vi "Area and time calculation_mains.vi"() -> ()   [LabVIEW 2014]
doc: "This example shows how to open, read, and display an AVI file in NI Vision. The VI reads the frames per second property and plays the images back at the rate specified by the AVI file."
uses:
  <vilib>/vision/NI_Vision_Development_Module.lvlib
panel:
  in  "Number of Erosion":i32=2
  in  "Low Pass/High Pass (Low)":bool
  out "t":dbl[][](array[numeric])
  out "s":dbl[][](array[numeric])
  in  "Info":bool
  in  "Binary":bool
  out "sum elements of array":dbl
  out "max value":dbl
  out "min value":dbl
  out "Error information":string
  out "Error of Velocity":dbl format="%#_4e"
  out "Velocity Mean":dbl format="%#_4e"
  out "Velocity\nArray":dbl[][](array[numeric])
  out "Y Step":sgl
  out "Num Final \nFrame":i32[](array[numeric])
  out "Num Initial\nFrame":i32[](array[numeric])
  in  "Velocity\nArray size":i32(slide)=3 scale=0.0..10.0
  in  "Range":cluster{"Lower value":sgl, "Upper value":sgl}={"Lower value"=0.0, "Upper value"=70.0}
  out "Initial Frame Pixel":dbl[](array[numeric])
  out "Initial Frame  Area":dbl[](array[numeric])
  out "Final Frame Area":dbl[](array[numeric])
  out "Final Frame Pixel":dbl[](array[numeric])
  out "pixel  value":dbl
  out "Area,µm^2":dbl
  in  "Si 2":T1={"X Size"=3, "Y Size"=3, "Order #"=4}
  out "appended array":i32[](array[numeric])
  out "dy":i32
  in  "Final Frame":i32(slide) scale=0.0..131.0
  in  "Initial Frame":i32(slide) scale=0.0..131.0
  out "time\nper frame":dbl
  in  "Frame":i32(slide) min=0 max=357 scale=0.0..131.0
  in  "Analyse":bool
  out "Image":T2(plugin-control)
  in  "stop":bool
  in  "Play":bool=TRUE
  # "White domain:\nRange 185-255"
  # "Black domain:\nRange 0-70"
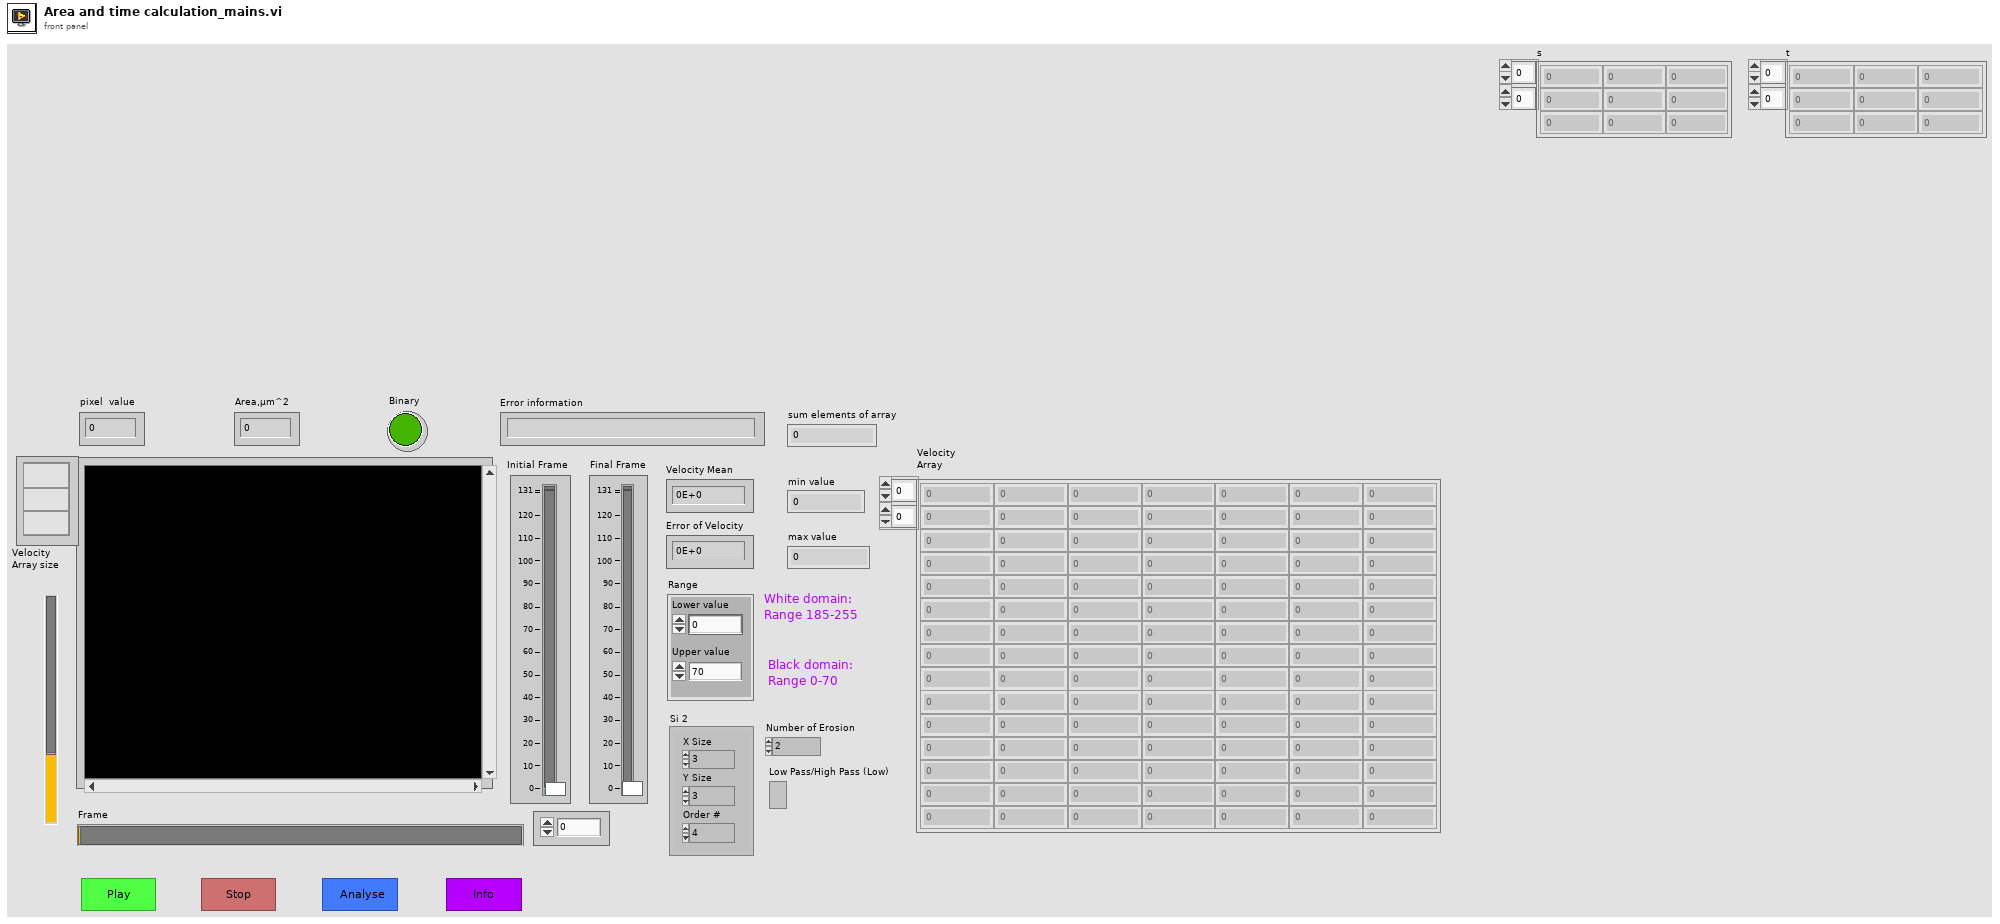
[diagram p1: front panel]
types:
  T1 = cluster{"X Size":i32, "Y Size":i32, "Order #":i32}
  T2 = typedef "IMAQ Image.ctl" = refnum<image>
  T3 = typedef "Image Type" = u32
  T4 = typedef "IMAQ AVI2 Refnum.ctl" = refnum<k20>
  T5 = cluster{"Width":u32, "Height":u32, "Frames Per Second":u32, "Codec":string, "Has Data":bool}
  T6 = typedef "Simple Grid Descriptor" = cluster{"X Step":sgl, "Y Step":sgl, "Unit":T7}
  T7 = typedef "Image Unit" = enum32{"Undefined", "Angström", "Micrometer", "Millimeter", "Centimeter", "Meter", "Kilometer", "Microinch", "Inch", "Feet", "Nautical miles", "Standard miles", "Steps"}
  T8 = cluster{"Global Rectangle":i32[], "Contours":cluster{"Contour Type":u32, "ROI Type":u32, "Points":i32[]}[]}
  T9 = typedef "IMAQ Rectangle" = cluster{"Left":i32, "Top":i32, "Right":i32, "Bottom":i32, "Rotation":dbl}
  T10 = typedef "Particle Parameters" = i32
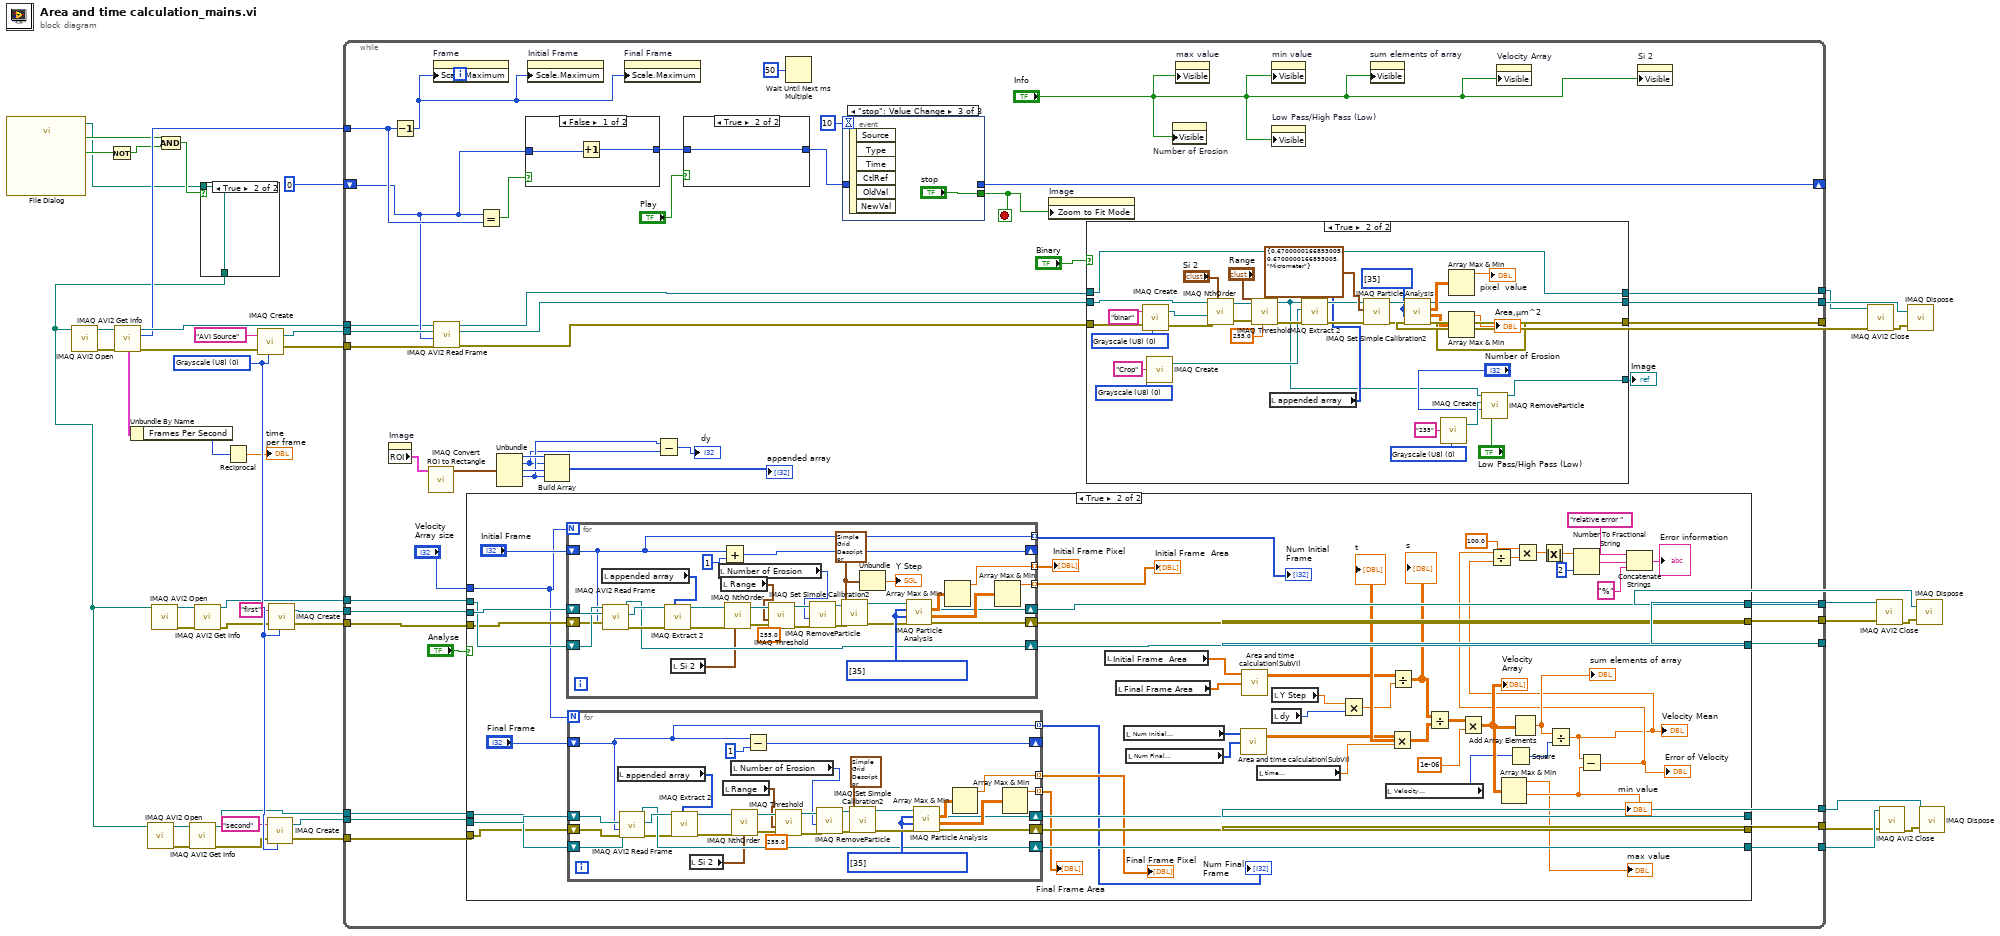
[diagram p0: block diagram]
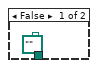
[diagram p2: hidden frame]
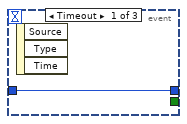
[diagram p4: hidden frame]
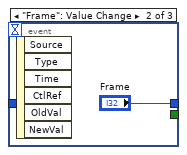
[diagram p5: hidden frame]
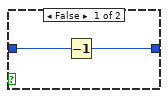
[diagram p7: hidden frame]
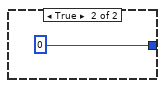
[diagram p8: hidden frame]
diagram:
  w37 = T3 0 items=["Grayscale (U8)", "Grayscale (I16)", "Grayscale (SGL)", "Complex (CSG)", "RGB (U32)", "HSL (U32)", "RGB (U64)", "Grayscale (U16)"] ("Image Type")
  n1 = call "File Dialog"() -> ("selected path"=w18:path, "exists"=w22:bool, "cancelled"=w21:bool)  [unwired: 12 in, 1 out]
  n2 = Not(x=w21) -> (.not. x?=w20:bool)
  n3 = Compound Arithmetic op=AND(w22, w20) -> (w19:bool)
  n4 = case shown="True" w19 {
    tunnel: w18 -> [_ w47]
    tunnel: [path "" ("selected path") w47] -> w6
    frame False {
    }
    frame True {
    }
  }
  n5 = call "IMAQ AVI2 Open"("AVI File Path"=w6) -> ("error out"=w45:errorcluster, "AVI Refnum"=w44:T4)  [unwired: 2 in, 7 out]
  n6 = call "IMAQ AVI2 Get Info"("error in (no error)"=w45, "AVI Refnum"=w44) -> ("error out"=w43:errorcluster, "Number of Frames"=w39:u32, "AVI Refnum (duplicate)"=w40:T4, "Frame Data"=w25:T5)  [unwired: 6 out]
  n7 = Unbundle By Name(w25) -> ("Frames Per Second"=w24:u32)
  n8 = call "IMAQ AVI2 Open"("AVI File Path"=w6) -> ("error out"=w33:errorcluster, "AVI Refnum"=w31:T4)  [unwired: 2 in, 7 out]
  n9 = call "IMAQ AVI2 Open"("AVI File Path"=w6) -> ("error out"=w34:errorcluster, "AVI Refnum"=w32:T4)  [unwired: 2 in, 7 out]
  n10 = call "IMAQ AVI2 Get Info"("error in (no error)"=w33, "AVI Refnum"=w31) -> ("error out"=w28:errorcluster, "AVI Refnum (duplicate)"=w16:T4)  [unwired: 8 out]
  n11 = call "IMAQ AVI2 Get Info"("error in (no error)"=w34, "AVI Refnum"=w32) -> ("error out"=w27:errorcluster, "AVI Refnum (duplicate)"=w26:T4)  [unwired: 8 out]
  n12 = Reciprocal(x=w24) -> (1/x=→"time\nper frame":dbl)
  n13 = call "IMAQ Create"("Image Name"="AVI Source", "Image Type"=w37, "error in (no error)"=w43) -> ("New Image"=w41:T2, "error out"=w42:errorcluster)  [unwired: 1 in, 1 out]
  n14 = call "IMAQ Create"("Image Name"="second", "Image Type"=w37, "error in (no error)"=w28) -> ("New Image"=w35:T2, "error out"=w15:errorcluster)  [unwired: 1 in, 1 out]
  n15 = call "IMAQ Create"("Image Name"="first", "Image Type"=w37, "error in (no error)"=w27) -> ("New Image"=w36:T2, "error out"=w14:errorcluster)  [unwired: 1 in, 1 out]
  n16 = while {
    tunnel: w41 -> [w91]
    tunnel: [w60] -> w1
    tunnel: w42 -> [w89]
    tunnel: w40 -> [w65]
    tunnel: w39 -> [w83]
    tunnel: w36 -> [w55]
    tunnel: w35 -> [w53]
    tunnel: w26 -> [w56]
    shift-right: [w84] -> _
    shift-left: u32 0 -> [w77]
    tunnel: w16 -> [w54]
    tunnel: w15 -> [w52]
    tunnel: w14 -> [w57]
    tunnel: [w76] -> w13
    tunnel: [w70] -> w12
    tunnel: [w69] -> w2
    tunnel: [w75] -> w11
    tunnel: [w74] -> w10
    tunnel: [w73] -> w8
    tunnel: [w63] -> w4
    tunnel: [w64] -> w3
    stop <- w66 stop-if-true
    n17 = property on="Image" class="ImageControl"() -> ("ROI"=w81:T8)  [unwired: 2 in, 2 out]
    n18 = Decrement(x=w83) -> (x-1=w58:u32)
    n19 = call "IMAQ Convert ROI to Rectangle"("ROI Descriptor"=w81) -> ("Rectangle"=w78:T9)  [unwired: 8 in, 1 out]
    n20 = property on="Frame" class="Slide (strict)"("Scale.Maximum"=w58) -> ()  [unwired: 2 in, 2 out]
    n21 = call "IMAQ AVI2 Read Frame"("error in (no error)"=w89, "Frame Number"=w77, "Image"=w91, "AVI Refnum"=w65) -> ("error out"=w49:errorcluster, "Image Out"=w50:T2, "AVI Refnum (duplicate)"=w51:T4)  [unwired: 5 out]
    n22 = case shown="True" "Analyse" {
      tunnel: w55 -> [w138 w192]
      tunnel: w53 -> [w136 w191]
      tunnel: w56 -> [w140 w190]
      tunnel: w54 -> [w137 w189]
      tunnel: w52 -> [w135 w188]
      tunnel: w57 -> [w139 w187]
      tunnel: [w140 w186] -> w76
      tunnel: [w138 w185] -> w70
      tunnel: [w136 w184] -> w69
      tunnel: [w137 w183] -> w75
      tunnel: [w135 w182] -> w74
      tunnel: [w139 w181] -> w73
      tunnel: "Velocity\nArray size" -> [_ w174]
      frame False {
      }
      frame True {
        n23 = for {
          N: w174 -> [_]
          shift-right: [w241] -> w185
          shift-left: w192 -> [w257]
          shift-right: [w242] -> w186
          shift-left: w190 -> [w256]
          shift-right: [w240] -> w181
          shift-left: w187 -> [w255]
          shift-right: [w234] -> _
          shift-left: "Initial Frame" -> [w233]
          tunnel: [w238] -> w176 mode=indexing
          tunnel: [w237] -> w175 mode=indexing
          tunnel: [w233] -> w161 mode=indexing
          w230 = T6 {"X Step"=0.67, "Y Step"=0.67, "Unit"=enum."Undefined"} ("Pixel Distances")
          w254 = T10[] [35] items=["Center of Mass X", "Center of Mass Y", "First Pixel X", "First Pixel Y", "Bounding Rect Left", "Bounding Rect Top", "Bounding Rect Right", "Bounding Rect Bottom", "Max Feret Diameter Start X", "Max Feret Diameter Start Y", "Max Feret Diameter End X", "Max Feret Diameter End Y", "Max Horiz. Segment Length Left", "Max Horiz. Segment Length Right", "Max Horiz. Segment Length Row", "-", "Bounding Rect Width", "Bounding Rect Height", "Bounding Rect Diagonal", "Perimeter", "Convex Hull Perimeter", "Holes' Perimeter", "Max Feret Diameter", "Equivalent Ellipse Major Axis", "Equivalent Ellipse Minor Axis", "Equivalent Ellipse Minor Axis (Feret)", "Equivalent Rect Long Side", "Equivalent Rect Short Side", "Equivalent Rect Diagonal", "Equivalent Rect Short Side (Feret)", "Average Horiz. Segment Length", "Average Vert. Segment Length", "Hydraulic Radius", "Waddel Disk Diameter", "-", "Area", "Holes' Area", "Particle & Holes' Area", "Convex Hull Area", "Image Area", "-", "Number of Holes", "Number of Horiz. Segments", "Number of Vert. Segments", "-", "Orientation", "Max Feret Diameter Orientation", "-", "% Area/Image Area", "% Area/(Particle & Holes' Area)", "Ratio of Equivalent Ellipse Axes", "Ratio of Equivalent Rect Sides", "-", "Elongation Factor", "Compactness Factor", "Heywood Circularity Factor", "Type Factor", "-", "Sum X", "Sum Y", "Sum XX", "Sum XY", "Sum YY", "Sum XXX", "Sum XXY", "Sum XYY", "Sum YYY", "-", "Moment of Inertia XX", "Moment of Inertia XY", "Moment of Inertia YY", "Moment of Inertia XXX", "Moment of Inertia XXY", "Moment of Inertia XYY", "Moment of Inertia YYY", "Norm. Moment of Inertia XX", "Norm. Moment of Inertia XY", "Norm. Moment of Inertia YY", "Norm. Moment of Inertia XXX", "Norm. Moment of Inertia XXY", "Norm. Moment of Inertia XYY", "Norm. Moment of Inertia YYY", "Hu Moment 1", "Hu Moment 2", "Hu Moment 3", "Hu Moment 4", "Hu Moment 5", "Hu Moment 6", "Hu Moment 7"] ("Pixel Measurements")
          n24 = local read "appended array"() -> (w235:i32[])
          n25 = call "IMAQ AVI2 Read Frame"("error in (no error)"=w255, "Frame Number"=w233, "Image"=w257, "AVI Refnum"=w256) -> ("error out"=w245:errorcluster, "Image Out"=w249:T2, "AVI Refnum (duplicate)"=w242:T4)  [unwired: 5 out]
          n26 = call "IMAQ Extract 2"("Optional Rectangle"=w235, "error in (no error)"=w245, "Image Src"=w249) -> ("error out"=w244:errorcluster, "Image Dst Out"=w248:T2)  [unwired: 7 in]
          n27 = local read "Si 2"() -> (w236:T1)
          n28 = local read "Number of Erosion"() -> (w225:i32)
          n29 = local read "Range"() -> (w231:cluster{"Lower value":sgl, "Upper value":sgl})
          n30 = Add(x=w233, y=1) -> (x+y=w234:i32)
          n31 = call "IMAQ NthOrder"("Image Src"=w248, "Size & Order #"=w236, "error in (no error)"=w244) -> ("Image Dst Out"=w247:T2, "error out"=w252:errorcluster)  [unwired: 4 in]
          n32 = call "IMAQ Threshold"("Replace Value"=sgl 255.0, "error in (no error)"=w252, "Range"=w231, "Image Src"=w247) -> ("error out"=w227:errorcluster, "Image Dst Out"=w229:T2)  [unwired: 6 in]
          n33 = call "IMAQ RemoveParticle"("error in (no error)"=w227, "Number of Erosion"=w225, "Image Src"=w229) -> ("error out"=w226:errorcluster, "Image Dst Out"=w228:T2)  [unwired: 7 in]
          n34 = call "IMAQ Set Simple Calibration2"("error in (no error)"=w226, "Pixel Distances"=w230, "Image"=w228) -> ("error out"=w243:errorcluster, "Calibration Template Image"=w246:T2)  [unwired: 7 in]
          n35 = Unbundle(w230) -> ("Y Step"=→"Y Step":sgl)  [unwired: 2 out]
          n36 = call "IMAQ Particle Analysis"("error in (no error)"=w243, "Real-World Measurements"=w254, "Pixel Measurements"=w254, "Image"=w246) -> ("error out"=w240:errorcluster, "Particle Measurements (Real-World)"=w250:dbl[][], "Particle Measurements (Pixels)"=w251:dbl[][], "Image Out (duplicate)"=w241:T2)  [unwired: 2 in, 2 out]
          n37 = Array Max & Min(array=w251) -> (max value=w238:dbl)  [unwired: 3 out]
          n38 = Array Max & Min(array=w250) -> (max value=w237:dbl)  [unwired: 3 out]
        }
        "Initial Frame Pixel" <- w176
        "Initial Frame  Area" <- w175
        "Num Initial\nFrame" <- w161
        n39 = for {
          N: w174 -> [_]
          shift-right: [w210] -> w184
          shift-left: w191 -> [w224]
          shift-right: [w209] -> w183
          shift-left: w189 -> [w223]
          shift-right: [w201] -> _
          shift-left: "Final Frame" -> [w200]
          tunnel: [w205] -> w178 mode=indexing
          tunnel: [w204] -> w177 mode=indexing
          shift-right: [w208] -> w182
          shift-left: w188 -> [w222]
          tunnel: [w200] -> w160 mode=indexing
          w212 = T10[] [35] items=["Center of Mass X", "Center of Mass Y", "First Pixel X", "First Pixel Y", "Bounding Rect Left", "Bounding Rect Top", "Bounding Rect Right", "Bounding Rect Bottom", "Max Feret Diameter Start X", "Max Feret Diameter Start Y", "Max Feret Diameter End X", "Max Feret Diameter End Y", "Max Horiz. Segment Length Left", "Max Horiz. Segment Length Right", "Max Horiz. Segment Length Row", "-", "Bounding Rect Width", "Bounding Rect Height", "Bounding Rect Diagonal", "Perimeter", "Convex Hull Perimeter", "Holes' Perimeter", "Max Feret Diameter", "Equivalent Ellipse Major Axis", "Equivalent Ellipse Minor Axis", "Equivalent Ellipse Minor Axis (Feret)", "Equivalent Rect Long Side", "Equivalent Rect Short Side", "Equivalent Rect Diagonal", "Equivalent Rect Short Side (Feret)", "Average Horiz. Segment Length", "Average Vert. Segment Length", "Hydraulic Radius", "Waddel Disk Diameter", "-", "Area", "Holes' Area", "Particle & Holes' Area", "Convex Hull Area", "Image Area", "-", "Number of Holes", "Number of Horiz. Segments", "Number of Vert. Segments", "-", "Orientation", "Max Feret Diameter Orientation", "-", "% Area/Image Area", "% Area/(Particle & Holes' Area)", "Ratio of Equivalent Ellipse Axes", "Ratio of Equivalent Rect Sides", "-", "Elongation Factor", "Compactness Factor", "Heywood Circularity Factor", "Type Factor", "-", "Sum X", "Sum Y", "Sum XX", "Sum XY", "Sum YY", "Sum XXX", "Sum XXY", "Sum XYY", "Sum YYY", "-", "Moment of Inertia XX", "Moment of Inertia XY", "Moment of Inertia YY", "Moment of Inertia XXX", "Moment of Inertia XXY", "Moment of Inertia XYY", "Moment of Inertia YYY", "Norm. Moment of Inertia XX", "Norm. Moment of Inertia XY", "Norm. Moment of Inertia YY", "Norm. Moment of Inertia XXX", "Norm. Moment of Inertia XXY", "Norm. Moment of Inertia XYY", "Norm. Moment of Inertia YYY", "Hu Moment 1", "Hu Moment 2", "Hu Moment 3", "Hu Moment 4", "Hu Moment 5", "Hu Moment 6", "Hu Moment 7"] ("Pixel Measurements")
          n40 = local read "appended array"() -> (w202:i32[])
          n41 = call "IMAQ AVI2 Read Frame"("error in (no error)"=w222, "Frame Number"=w200, "Image"=w224, "AVI Refnum"=w223) -> ("error out"=w207:errorcluster, "Image Out"=w211:T2, "AVI Refnum (duplicate)"=w209:T4)  [unwired: 5 out]
          n42 = call "IMAQ Extract 2"("Optional Rectangle"=w202, "error in (no error)"=w207, "Image Src"=w211) -> ("error out"=w220:errorcluster, "Image Dst Out"=w217:T2)  [unwired: 7 in]
          n43 = local read "Si 2"() -> (w203:T1)
          n44 = local read "Range"() -> (w199:cluster{"Lower value":sgl, "Upper value":sgl})
          n45 = local read "Number of Erosion"() -> (w193:i32)
          n46 = call "IMAQ NthOrder"("Image Src"=w217, "Size & Order #"=w203, "error in (no error)"=w220) -> ("Image Dst Out"=w218:T2, "error out"=w214:errorcluster)  [unwired: 4 in]
          n47 = Subtract(x=w200, y=1) -> (x-y=w201:i32)
          n48 = call "IMAQ Threshold"("Replace Value"=sgl 255.0, "error in (no error)"=w214, "Range"=w199, "Image Src"=w218) -> ("error out"=w197:errorcluster, "Image Dst Out"=w196:T2)  [unwired: 6 in]
          n49 = call "IMAQ RemoveParticle"("error in (no error)"=w197, "Number of Erosion"=w193, "Image Src"=w196) -> ("error out"=w194:errorcluster, "Image Dst Out"=w195:T2)  [unwired: 7 in]
          n50 = call "IMAQ Set Simple Calibration2"("error in (no error)"=w194, "Pixel Distances"=T6 {"X Step"=0.67, "Y Step"=0.67, "Unit"=enum."Micrometer"}, "Image"=w195) -> ("error out"=w221:errorcluster, "Calibration Template Image"=w219:T2)  [unwired: 7 in]
          n51 = call "IMAQ Particle Analysis"("error in (no error)"=w221, "Real-World Measurements"=w212, "Pixel Measurements"=w212, "Image"=w219) -> ("error out"=w208:errorcluster, "Particle Measurements (Real-World)"=w216:dbl[][], "Particle Measurements (Pixels)"=w215:dbl[][], "Image Out (duplicate)"=w210:T2)  [unwired: 2 in, 2 out]
          n52 = Array Max & Min(array=w215) -> (max value=w205:dbl)  [unwired: 3 out]
          n53 = Array Max & Min(array=w216) -> (max value=w204:dbl)  [unwired: 3 out]
        }
        "Final Frame Pixel" <- w178
        "Final Frame Area" <- w177
        "Num Final \nFrame" <- w160
        n54 = local read "Initial Frame  Area"() -> (w142:dbl[])
        n55 = local read "Final Frame Area"() -> (w143:dbl[])
        n56 = local read "Num Initial\nFrame"() -> (w162:i32[])
        n57 = local read "Num Final \nFrame"() -> (w163:i32[])
        n58 = call "Area and time calculation(SubVI).vi"("Array in 2"=w163, "Array in"=w162) -> ("Array out"=w164:dbl[][])  [unwired: 2 in]
        n59 = call "Area and time calculation(SubVI).vi"("Array in 2"=w143, "Array in"=w142) -> ("Array out"=w168:dbl[][])  [unwired: 2 in]
        n60 = local read "time\nper frame"() -> (w165:dbl)
        n61 = local read "Y Step"() -> (w166:sgl)
        n62 = local read "dy"() -> (w167:i32)
        n63 = Multiply(x=w166, y=w167) -> (x*y=w169:sgl)
        n64 = local read "Velocity\nArray size"() -> (w149:i32)
        n65 = Multiply(x=w164, y=w165) -> (x*y=w171:dbl[][])
        "t" <- w171
        n66 = Divide(x=w168, y=w169) -> (x/y=w170:dbl[][])
        "s" <- w170
        n67 = Divide(x=w170, y=w171) -> (x/y=w172:dbl[][])
        n68 = Multiply(x=w172, y=1e-06) -> (x*y=w159:dbl[][])
        "Velocity\nArray" <- w159
        n69 = Array Max & Min(array=w159) -> (max value=→"max value":dbl, min value=w157:dbl)  [unwired: 2 out]
        "min value" <- w157
        n70 = Square(x=w149) -> (x^2=w148:i32)
        n71 = Add Array Elements(numeric array=w159) -> (sum=w158:dbl)
        "sum elements of array" <- w158
        n72 = Divide(x=w158, y=w148) -> (x/y=w146:dbl)
        "Velocity Mean" <- w146
        n73 = Subtract(x=w146, y=w157) -> (x-y=w147:dbl)
        "Error of Velocity" <- w147
        n74 = Divide(x=w147, y=w146) -> (x/y=w156:dbl)
        n75 = Multiply(x=100.0, y=w156) -> (x*y=w145:dbl)
        n76 = Absolute Value(x=w145) -> (abs(x)=w144:dbl)
        n77 = Number To Fractional String(number=w144, precision (6)=i16 2) -> (F-format string=w154:string)  [unwired: 2 in]
        n78 = Concatenate Strings("relative error " ("string"), w154, "%" ("string")) -> (→"Error information":string)
      }
    }
    n79 = Equal?(x=w77, y=w83) -> (x = y?=w92:bool)
    n80 = Unbundle(w78) -> ("Left"=w80:i32, "Top"=w67:i32, "Right"=w79:i32, "Bottom"=w68:i32)  [unwired: 1 out]
    n81 = case shown="False" w92 {
      tunnel: w77 -> [w262 _]
      tunnel: [w261 i16 0] -> w86
      frame False {
        n82 = Increment(x=w262) -> (x+1=w261:u32)
      }
      frame True {
      }
    }
    n83 = property on="Initial Frame" class="Slide (strict)"("Scale.Maximum"=w58) -> ()  [unwired: 2 in, 2 out]
    n84 = Build Array(w80, w67, w79, w68) -> (→"appended array":i32[])
    n85 = property on="Final Frame" class="Slide (strict)"("Scale.Maximum"=w58) -> ()  [unwired: 2 in, 2 out]
    n86 = Subtract(x=w68, y=w67) -> (x-y=→"dy":i32)
    n87 = case shown="True" "Play" {
      tunnel: w86 -> [w259 w260]
      tunnel: [w258 w260] -> w85
      frame False {
        n88 = Decrement(x=w259) -> (x-1=w258:u32)
      }
      frame True {
      }
    }
    n89 = Wait Until Next ms Multiple(millisecond multiple=u32 50) -> ()  [unwired: 1 out]
    n90 = event shown="[2] \"stop\": Value Change" {
      selector: _ -> [_ _ _]
      dyn-events: _ -> [_ _ _]
      timeout: 10 -> [_ _ _]
      tunnel: w85 -> [w132 _ _]
      tunnel: [w132 "Frame" _] -> w84
      tunnel: [_ _ "stop"] -> w66
      event Timeout {
        n91 = event-data() -> ()  [unwired: 1 in, 3 out]
      }
      event "Frame": Value Change {
        n92 = event-data() -> ()  [unwired: 1 in, 6 out]
      }
      event "stop": Value Change {
        n93 = event-data() -> ()  [unwired: 1 in, 6 out]
      }
    }
    n94 = property on="Image" class="ImageControl"("Zoom to Fit Mode"=w66) -> ()  [unwired: 2 in, 2 out]
    n95 = case shown="True" "Binary" {
      tunnel: w51 -> [w95 w117]
      tunnel: [w95 w117] -> w60
      tunnel: w49 -> [w94 w128]
      tunnel: w50 -> [w93 w111]
      tunnel: [w93 w118] -> w63
      tunnel: [w94 w114] -> w64
      tunnel: [w93 w102] -> w61
      frame False {
      }
      frame True {
        w97 = T3 0 items=["Grayscale (U8)", "Grayscale (I16)", "Grayscale (SGL)", "Complex (CSG)", "RGB (U32)", "HSL (U32)", "RGB (U64)", "Grayscale (U16)"] ("Image Type")
        w104 = T3 0 items=["Grayscale (U8)", "Grayscale (I16)", "Grayscale (SGL)", "Complex (CSG)", "RGB (U32)", "HSL (U32)", "RGB (U64)", "Grayscale (U16)"] ("Image Type")
        w121 = T10[] [35] items=["Center of Mass X", "Center of Mass Y", "First Pixel X", "First Pixel Y", "Bounding Rect Left", "Bounding Rect Top", "Bounding Rect Right", "Bounding Rect Bottom", "Max Feret Diameter Start X", "Max Feret Diameter Start Y", "Max Feret Diameter End X", "Max Feret Diameter End Y", "Max Horiz. Segment Length Left", "Max Horiz. Segment Length Right", "Max Horiz. Segment Length Row", "-", "Bounding Rect Width", "Bounding Rect Height", "Bounding Rect Diagonal", "Perimeter", "Convex Hull Perimeter", "Holes' Perimeter", "Max Feret Diameter", "Equivalent Ellipse Major Axis", "Equivalent Ellipse Minor Axis", "Equivalent Ellipse Minor Axis (Feret)", "Equivalent Rect Long Side", "Equivalent Rect Short Side", "Equivalent Rect Diagonal", "Equivalent Rect Short Side (Feret)", "Average Horiz. Segment Length", "Average Vert. Segment Length", "Hydraulic Radius", "Waddel Disk Diameter", "-", "Area", "Holes' Area", "Particle & Holes' Area", "Convex Hull Area", "Image Area", "-", "Number of Holes", "Number of Horiz. Segments", "Number of Vert. Segments", "-", "Orientation", "Max Feret Diameter Orientation", "-", "% Area/Image Area", "% Area/(Particle & Holes' Area)", "Ratio of Equivalent Ellipse Axes", "Ratio of Equivalent Rect Sides", "-", "Elongation Factor", "Compactness Factor", "Heywood Circularity Factor", "Type Factor", "-", "Sum X", "Sum Y", "Sum XX", "Sum XY", "Sum YY", "Sum XXX", "Sum XXY", "Sum XYY", "Sum YYY", "-", "Moment of Inertia XX", "Moment of Inertia XY", "Moment of Inertia YY", "Moment of Inertia XXX", "Moment of Inertia XXY", "Moment of Inertia XYY", "Moment of Inertia YYY", "Norm. Moment of Inertia XX", "Norm. Moment of Inertia XY", "Norm. Moment of Inertia YY", "Norm. Moment of Inertia XXX", "Norm. Moment of Inertia XXY", "Norm. Moment of Inertia XYY", "Norm. Moment of Inertia YYY", "Hu Moment 1", "Hu Moment 2", "Hu Moment 3", "Hu Moment 4", "Hu Moment 5", "Hu Moment 6", "Hu Moment 7"] ("Pixel Measurements")
        w129 = T3 0 items=["Grayscale (U8)", "Grayscale (I16)", "Grayscale (SGL)", "Complex (CSG)", "RGB (U32)", "HSL (U32)", "RGB (U64)", "Grayscale (U16)"] ("Image Type")
        n96 = call "IMAQ Create"("Image Name"="binar", "Image Type"=w129, "error in (no error)"=w128) -> ("New Image"=w112:T2, "error out"=w110:errorcluster)  [unwired: 1 in, 1 out]
        n97 = call "IMAQ Create"("Image Name"="Crop", "Image Type"=w104) -> ("New Image"=w103:T2)  [unwired: 2 in, 2 out]
        n98 = call "IMAQ NthOrder"("Image Src"=w111, "Size & Order #"="Si 2", "Image Dst"=w112, "error in (no error)"=w110) -> ("Image Dst Out"=w131:T2, "error out"=w127:errorcluster)  [unwired: 3 in]
        n99 = call "IMAQ Threshold"("Replace Value"=sgl 255.0, "error in (no error)"=w127, "Range"="Range", "Image Src"=w131) -> ("error out"=w109:errorcluster, "Image Dst Out"=w96:T2)  [unwired: 6 in]
        n100 = local read "appended array"() -> (w106:i32[])
        n101 = call "IMAQ Extract 2"("Optional Rectangle"=w106, "error in (no error)"=w109, "Image Dst"=w103, "Image Src"=w96) -> ("error out"=w108:errorcluster, "Image Dst Out"=w107:T2)  [unwired: 6 in]
        n102 = call "IMAQ Set Simple Calibration2"("error in (no error)"=w108, "Pixel Distances"=T6 {"X Step"=0.67, "Y Step"=0.67, "Unit"=enum."Micrometer"}, "Image"=w107) -> ("error out"=w123:errorcluster, "Calibration Template Image"=w122:T2)  [unwired: 7 in]
        n103 = call "IMAQ Particle Analysis"("error in (no error)"=w123, "Real-World Measurements"=w121, "Pixel Measurements"=w121, "Image"=w122) -> ("error out"=w114:errorcluster, "Particle Measurements (Real-World)"=w119:dbl[][], "Particle Measurements (Pixels)"=w120:dbl[][], "Image Out (duplicate)"=w118:T2)  [unwired: 2 in, 2 out]
        n104 = call "IMAQ Create"("Image Name"="235", "Image Type"=w97) -> ("New Image"=w101:T2)  [unwired: 2 in, 2 out]
        n105 = Array Max & Min(array=w120) -> (max value=→"pixel  value":dbl)  [unwired: 3 out]
        n106 = Array Max & Min(array=w119) -> (max value=→"Area,µm^2":dbl)  [unwired: 3 out]
        n107 = call "IMAQ RemoveParticle"("Low Pass/High Pass (Low)"="Low Pass/High Pass (Low)", "Number of Erosion"="Number of Erosion", "Image Dst"=w101, "Image Src"=w96) -> ("Image Dst Out"=w102:T2)  [unwired: 6 in, 1 out]
      }
    }
    "Image" <- w61
    n108 = property on="Number of Erosion" class="DigNum (strict)"("Visible"="Info") -> ()  [unwired: 2 in, 2 out]
    n109 = property on="max value" class="DigNum (strict)"("Visible"="Info") -> ()  [unwired: 2 in, 2 out]
    n110 = property on="min value" class="DigNum (strict)"("Visible"="Info") -> ()  [unwired: 2 in, 2 out]
    n111 = property on="Low Pass/High Pass (Low)" class="Bool (strict)"("Visible"="Info") -> ()  [unwired: 2 in, 2 out]
    n112 = property on="sum elements of array" class="DigNum (strict)"("Visible"="Info") -> ()  [unwired: 2 in, 2 out]
    n113 = property on="Velocity Array" class="Arr (strict)"("Visible"="Info") -> ()  [unwired: 2 in, 2 out]
    n114 = property on="Si 2" class="Clust (strict)"("Visible"="Info") -> ()  [unwired: 2 in, 2 out]
  }
  n115 = call "IMAQ AVI2 Close"("error in (no error)"=w3, "AVI Refnum"=w1) -> ("error out"=w5:errorcluster)  [unwired: 9 out]
  n116 = call "IMAQ AVI2 Close"("error in (no error)"=w8, "AVI Refnum"=w13) -> ("error out"=w7:errorcluster)  [unwired: 9 out]
  n117 = call "IMAQ AVI2 Close"("error in (no error)"=w10, "AVI Refnum"=w11) -> ("error out"=w9:errorcluster)  [unwired: 9 out]
  n118 = call "IMAQ Dispose"("Image"=w4, "error in (no error)"=w5) -> ()  [unwired: 1 in, 4 out]
  n119 = call "IMAQ Dispose"("Image"=w12, "error in (no error)"=w7) -> ()  [unwired: 1 in, 4 out]
  n120 = call "IMAQ Dispose"("Image"=w2, "error in (no error)"=w9) -> ()  [unwired: 1 in, 4 out]
